vi "Movement_Picture_ClusterInput.vi"(11 "Oculus Data out":T1) -> (3 "2D Picture":picture)   [LabVIEW 2017]
panel:
  in  "rect":T2={"left"=0, "top"=0, "right"=407, "bottom"=407}
  out "output cluster 2":cluster{dbl, dbl}={149.4878, 198.5598}
  in  "Arrow Size":dbl=15.0 format="%#_13g"
  in  "Rotation Radius":dbl=50.0 format="%#_13g"
  out "output cluster":cluster{dbl, dbl}={199.4878, 198.5598}
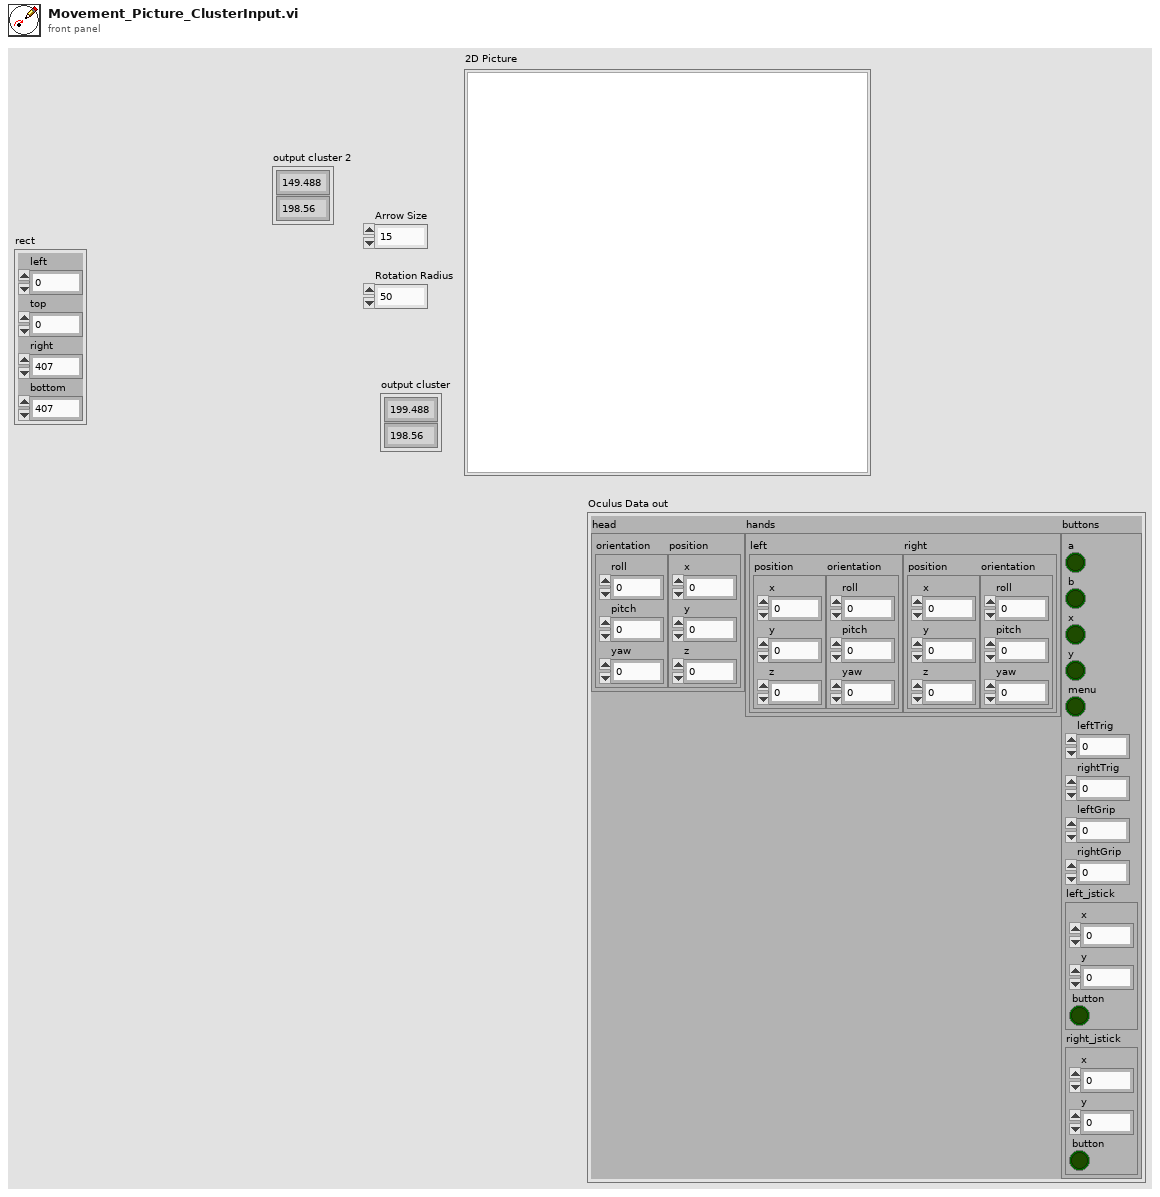
[diagram p1: front panel]
types:
  T1 = cluster{"head":cluster{"orientation":cluster{"roll":dbl, "pitch":dbl, "yaw":dbl}, "position":cluster{"x":dbl, "y":dbl, "z":dbl}}, "hands":cluster{"left":cluster{"position":cluster{"x":dbl, "y":dbl, "z":dbl}, "orientation":cluster{"roll":dbl, "pitch":dbl, "yaw":dbl}}, "right":cluster{"position":cluster{"x":dbl, "y":dbl, "z":dbl}, "orientation":cluster{"roll":dbl, "pitch":dbl, "yaw":dbl}}}, "buttons":cluster{"a":bool, "b":bool, "x":bool, "y":bool, "menu":bool, "leftTrig":dbl, "rightTrig":dbl, "leftGrip":dbl, "rightGrip":dbl, "left_jstick":cluster{"x":dbl, "y":dbl, "button":bool}, "right_jstick":cluster{"x":dbl, "y":dbl, "button":bool}}}
  T2 = cluster{"left":i16, "top":i16, "right":i16, "bottom":i16}
  T3 = cluster{"Width":u16, "Style":enum32{"Solid", "Dash", "Dot", "DashDot", "DashDotDot"}}
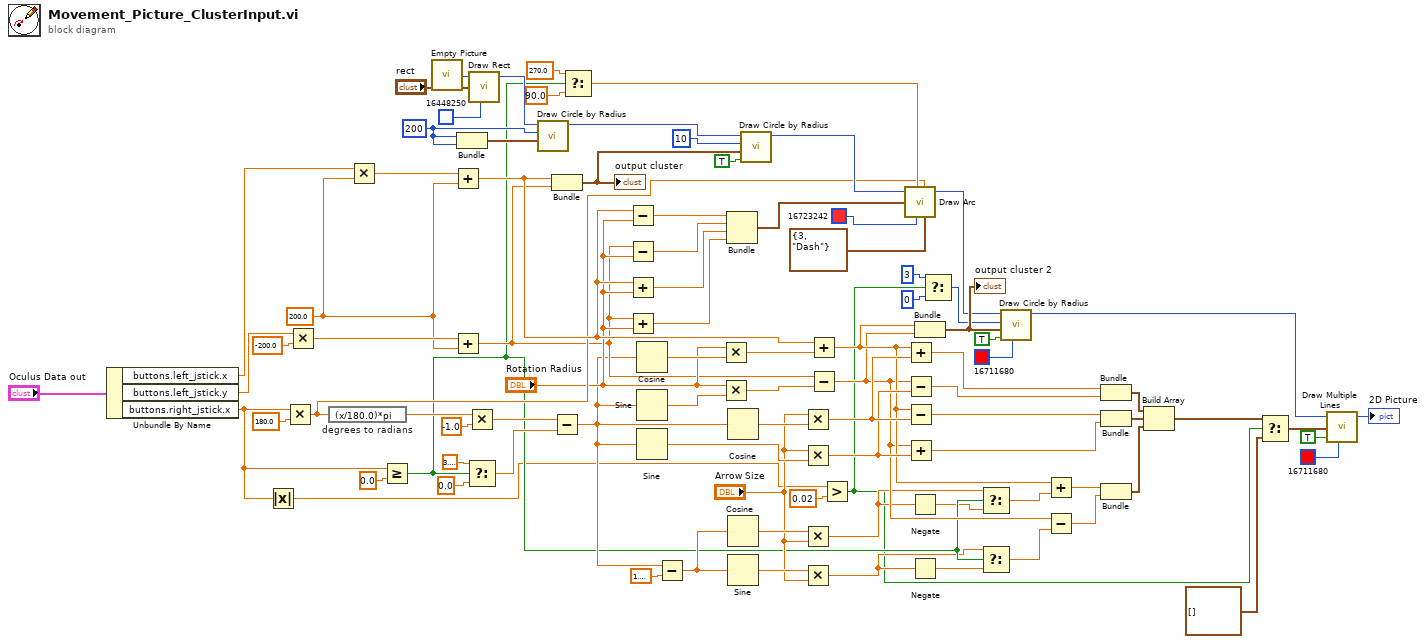
[diagram p0: block diagram]
diagram:
  w85 = 200.0 ("y")
  w90 = i16 200 ("radius")
  n1 = Unbundle By Name("Oculus Data out") -> ("buttons.left_jstick.x"=w2:dbl, "buttons.left_jstick.y"=w1:dbl, "buttons.right_jstick.x"=w3:dbl)
  n2 = Absolute Value(x=w3) -> (abs(x)=w13:dbl)
  n3 = Multiply(x=w3, y=180.0) -> (x*y=w42:dbl)
  n4 = Multiply(x=w1, y=-200.0) -> (x*y=w87:dbl)
  n5 = expression code="(x/180.0)*pi" "degrees to radians"(w42) -> (w37:dbl)
  n6 = Multiply(x=w2, y=w85) -> (x*y=w88:dbl)
  n7 = Greater Or Equal?(x=w3, y=0.0) -> (x >= y?=w21:bool)
  n8 = call "Empty Picture"() -> ("empty picture"=w66:picture)
  n9 = Add(x=w88, y=w85) -> (x+y=w43:dbl)
  n10 = Add(x=w87, y=w85) -> (x+y=w34:dbl)
  n11 = Bundle("radius"=w90, "radius"=w90) -> (w89:cluster{"radius":i16, "radius":i16})  [unwired: 1 in]
  n12 = Multiply(x=w37, y=-1.0) -> (x*y=w35:dbl)
  n13 = Select(t=3.141592653589793, s=w21, f=0.0) -> (s? t:f=w24:dbl)
  n14 = call <vilib>:"Draw Rect.vi"("picture"=w66, "rect"="rect", "color(black)"=u32 16448250) -> ("new picture"=w67:picture)  [unwired: 6 in]
  n15 = call <vilib>:"Draw Circle by Radius.vi"("pixel center"=w89, "radius"=w90, "picture"=w67) -> ("new picture"=w84:picture)  [unwired: 8 in]
  n16 = Bundle(w43, w34) -> (w82:cluster{dbl, dbl})  [unwired: 1 in]
  "output cluster" <- w82
  n17 = Subtract(x=w35, y=w24) -> (x-y=w25:dbl)
  n18 = Select(t=270.0, s=w21, f=90.0) -> (s? t:f=w76:dbl)
  n19 = Subtract(x=w43, y="Rotation Radius") -> (x-y=w72:dbl)
  n20 = Subtract(x=w34, y="Rotation Radius") -> (x-y=w70:dbl)
  n21 = Add(x=w43, y="Rotation Radius") -> (x+y=w71:dbl)
  n22 = Add(x=w34, y="Rotation Radius") -> (x+y=w69:dbl)
  n23 = Cosine(x=w25) -> (cos(x)=w41:dbl)
  n24 = Sine(x=w25) -> (sin(x)=w40:dbl)
  n25 = Sine(x=w25) -> (sin(x)=w56:dbl)
  n26 = Subtract(x=w25, y=1.5707963267948966) -> (x-y=w49:dbl)
  n27 = Multiply(x="Rotation Radius", y=w41) -> (x*y=w38:dbl)
  n28 = Multiply(x="Rotation Radius", y=w40) -> (x*y=w33:dbl)
  n29 = Bundle(w72, w70, w71, w69) -> (w68:cluster{dbl, dbl, dbl, dbl})  [unwired: 1 in]
  n30 = Cosine(x=w25) -> (cos(x)=w62:dbl)
  n31 = Cosine(x=w49) -> (cos(x)=w47:dbl)
  n32 = Sine(x=w49) -> (sin(x)=w48:dbl)
  n33 = call <vilib>:"Draw Circle by Radius.vi"("fill?(F)"=TRUE, "pixel center"=w82, "radius"=i16 10, "picture"=w84) -> ("new picture"=w80:picture)  [unwired: 7 in]
  n34 = Multiply(x="Arrow Size", y=w62) -> (x*y=w54:dbl)
  n35 = Multiply(x="Arrow Size", y=w56) -> (x*y=w51:dbl)
  n36 = Multiply(x=w47, y="Arrow Size") -> (x*y=w15:dbl)
  n37 = Multiply(x=w48, y="Arrow Size") -> (x*y=w19:dbl)
  n38 = Add(x=w43, y=w38) -> (x+y=w31:dbl)
  n39 = Subtract(x=w34, y=w33) -> (x-y=w30:dbl)
  n40 = Greater?(x=w13, y=0.02 ("f")) -> (0:w11:bool)
  n41 = call <vilib>:"Draw Arc.vi"("picture"=w80, "start angle[degrees]"=w76, "rect"=w68, "color(black)"=u32 16723242, "arc size[degrees]"=w42, "pen"=T3 {"Width"=3, "Style"=enum."Dash"}) -> ("new picture"=w27:picture)  [unwired: 3 in]
  n42 = Add(x=w31, y=w54) -> (x+y=w57:dbl)
  n43 = Subtract(x=w30, y=w51) -> (x-y=w55:dbl)
  n44 = Subtract(x=w31, y=w54) -> (x-y=w53:dbl)
  n45 = Add(x=w30, y=w51) -> (x+y=w52:dbl)
  n46 = Negate(x=w15) -> (-x=w16:dbl)
  n47 = Negate(x=w19) -> (-x=w20:dbl)
  n48 = Bundle(w31, w30) -> (w29:cluster{dbl, dbl})  [unwired: 1 in]
  "output cluster 2" <- w29
  n49 = Select(t=i16 3 ("radius"), s=w11, f=i16 0) -> (s? t:f=w7:i16)
  n50 = Select(t=w15, s=w21, f=w16) -> (s? t:f=w17:dbl)
  n51 = Select(t=w19, s=w21, f=w20) -> (s? t:f=w18:dbl)
  n52 = call <vilib>:"Draw Circle by Radius.vi"("color(black)"=u32 16711680, "fill?(F)"=TRUE, "pixel center"=w29, "radius"=w7, "picture"=w27) -> ("new picture"=w28:picture)  [unwired: 6 in]
  n53 = Add(x=w31, y=w17) -> (x+y=w44:dbl)
  n54 = Subtract(x=w30, y=w18) -> (x-y=w45:dbl)
  n55 = Bundle(w57, w55) -> (w60:cluster{dbl, dbl})  [unwired: 1 in]
  n56 = Bundle(w53, w52) -> (w59:cluster{dbl, dbl})  [unwired: 1 in]
  n57 = Bundle(w44, w45) -> (w58:cluster{dbl, dbl})  [unwired: 1 in]
  n58 = Build Array(w60, w59, w58) -> (w10:cluster{dbl, dbl}[])
  n59 = Select(t=w10, s=w11, f=cluster{"x":i16, "y":i16}[] [] ("line endpoints")) -> (s? t:f=w8:cluster{"x":dbl, "y":dbl}[])
  n60 = call <vilib>:"Draw Multiple Lines.vi"("picture"=w28, "line endpoints"=w8, "fill?(F)"=TRUE, "color(black)"=u32 16711680) -> ("new picture"=→"2D Picture":picture)  [unwired: 5 in]
